vi "Receive.vi"(11 "Base Queue jettl in":refnum<class "Base Queue jettl.lvclass">) -> (2 "Msg Strategy":refnum<class "Msg Strategy.lvclass">, 3 "Base Queue jettl out":refnum<class "Base Queue jettl.lvclass">)   [LabVIEW 2021, in "jettl.lvlib" / "Base Queue jettl.lvlib" / "Base Queue jettl.lvclass"]
uses:
  Base Queue jettl.lvclass
  Msg Strategy/Msg Strategy.lvclass
  Base Queue jettl.lvclass/Base Queue jettl.ctl
  Self Queue/Self Queue.lvlib
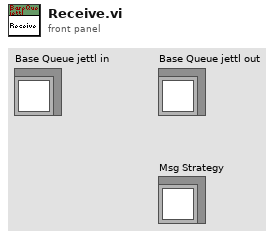
[diagram p1: front panel]
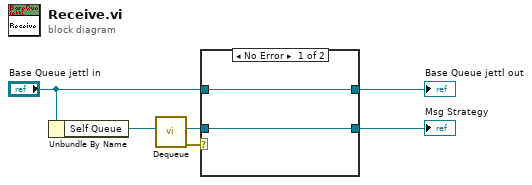
[diagram p0: block diagram]
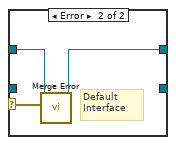
[diagram p2: hidden frame]
diagram:
  n1 = Unbundle By Name("Base Queue jettl in") -> ("Self Queue"=w3:refnum<data-value>)
  n2 = call "Dequeue.vi"("Self Queue"=w3) -> ("error out"=w2:errorcluster, "Msg Strategy"=w1:refnum<class "Msg Strategy.lvclass">)  [unwired: 9 in]
  n3 = case shown="No Error" w2 {
    selector: w2 -> [_ w9]
    tunnel: w1 -> [w7 _]
    tunnel: "Base Queue jettl in" -> [w8 w11]
    tunnel: [w8 w10] -> w6
    tunnel: [w7 _] -> w5
    frame No Error {
    }
    frame Error {
      # "Default Interface"
      n4 = call-dynamic "Merge Error.vi"("Error"=w9, "Base Queue jettl in"=w11) -> ("Base Queue jettl out"=w10:refnum<class "Base Queue jettl.lvclass">)  [unwired: 9 in]
    }
  }
  "Base Queue jettl out" <- w6
  "Msg Strategy" <- w5
